vi "Draw.vi"(8 "error in (no error)":errorcluster, 11 "Game Data in":T1) -> (0 "error out":errorcluster, 2 "Colors":u32[](array[colorbox]), 3 "Game Data out":T1)   [LabVIEW 2025]
uses:
  Game Data.ctl
  Bullet Data.ctl
  Game State.ctl
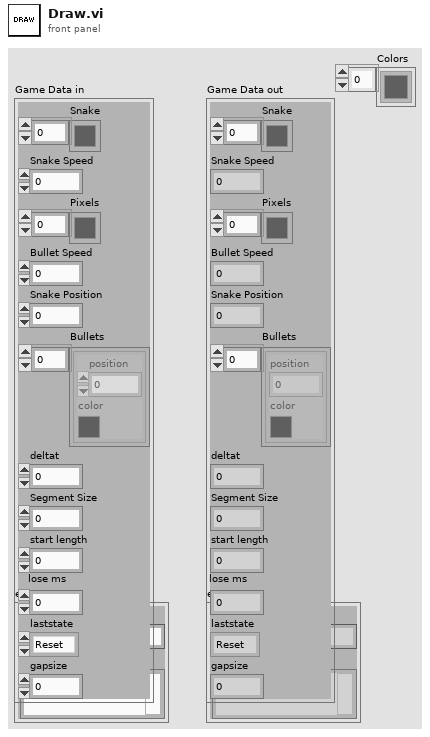
[diagram p1: front panel]
types:
  T1 = typedef "Game Data.ctl" = cluster{"Snake":u32[], "Snake Speed":dbl, "Pixels":u32[], "Bullet Speed":dbl, "Snake Position":dbl, "Bullets":T2[], "deltat":dbl, "Segment Size":dbl, "start length":u32, "lose ms":u32, "laststate":T3, "gapsize":i32}
  T2 = typedef "Bullet Data.ctl" = cluster{"position":dbl, "color":u32}
  T3 = typedef "Game State.ctl" = enum16{"Reset", "Idle", "Start", "Playing", "Win", "Lose"}
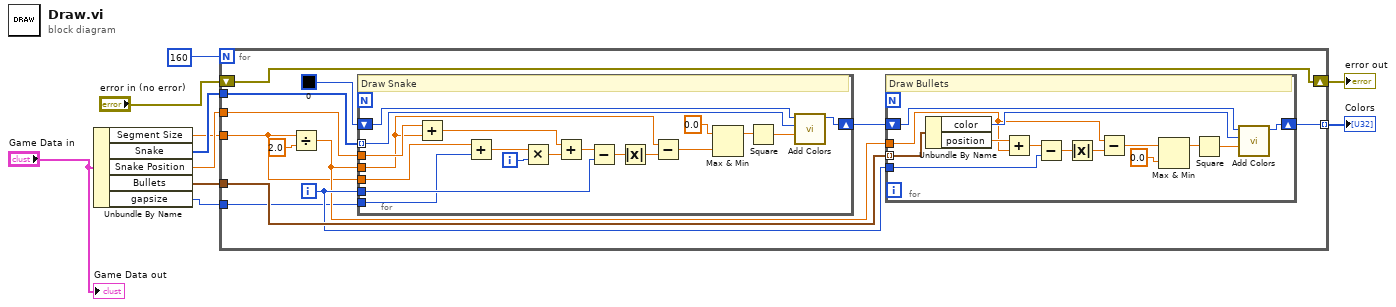
[diagram p0: block diagram]
diagram:
  n1 = Unbundle By Name("Game Data in") -> ("Segment Size"=w4:dbl, "Snake"=w6:u32[], "Snake Position"=w5:dbl, "Bullets"=w7:T2[], "gapsize"=w1:i32)
  n2 = for {
    N: 160 ("dimension size") -> [_]
    shift-right: [w22] -> w8
    shift-left: "error in (no error)" -> [w22]
    tunnel: w7 -> [w19]
    tunnel: w6 -> [w21]
    tunnel: w5 -> [w20]
    tunnel: [w14] -> w3 mode=indexing
    tunnel: w4 -> [w12]
    tunnel: w1 -> [w11]
    i -> [w18]
    n3 = Divide(x=w12, y=2.0) -> (x/y=w13:dbl)
    n4 = for {
      tunnel: w21 -> [w52] mode=indexing
      tunnel: w13 -> [w40]
      tunnel: w20 -> [w54]
      tunnel: w18 -> [w45]
      shift-right: [w49] -> w15
      shift-left: u32 0 ("Color out") -> [w50]
      tunnel: w12 -> [w42]
      tunnel: w11 -> [w37]
      i -> [w55]
      # "Draw Snake"
      n5 = Add(x=w54, y=w40) -> (x+y=w41:dbl)
      n6 = Add(x=w42, y=w37) -> (x+y=w43:dbl)
      n7 = Multiply(x=w43, y=w55) -> (x*y=w53:dbl)
      n8 = Add(x=w41, y=w53) -> (x+y=w46:dbl)
      n9 = Subtract(x=w46, y=w45) -> (x-y=w44:dbl)
      n10 = Absolute Value(x=w44) -> (abs(x)=w47:dbl)
      n11 = Subtract(x=w40, y=w47) -> (x-y=w51:dbl)
      n12 = Max & Min(x=0.0, y=w51) -> (max(x,y)=w39:dbl)  [unwired: 1 out]
      n13 = Square(x=w39) -> (x^2=w38:dbl)
      n14 = call "Add Colors.vi"("Factor (1)"=w38, "Color in"=w52, "color"=w50) -> ("Color out"=w49:u32)  [unwired: 8 in]
    }
    n15 = for {
      tunnel: w19 -> [w36] mode=indexing
      tunnel: w13 -> [w24]
      tunnel: w18 -> [w34]
      shift-right: [w29] -> w14
      shift-left: w15 -> [w28]
      # "Draw Bullets"
      n16 = Unbundle By Name(w36) -> ("color"=w27:u32, "position"=w35:dbl)
      n17 = Add(x=w35, y=w24) -> (x+y=w25:dbl)
      n18 = Subtract(x=w25, y=w34) -> (x-y=w33:dbl)
      n19 = Absolute Value(x=w33) -> (abs(x)=w32:dbl)
      n20 = Subtract(x=w24, y=w32) -> (x-y=w31:dbl)
      n21 = Max & Min(x=w31, y=0.0) -> (max(x,y)=w26:dbl)  [unwired: 1 out]
      n22 = Square(x=w26) -> (x^2=w23:dbl)
      n23 = call "Add Colors.vi"("Factor (1)"=w23, "Color in"=w27, "color"=w28) -> ("Color out"=w29:u32)  [unwired: 8 in]
    }
  }
  "error out" <- w8
  "Colors" <- w3
  "Game Data out" <- "Game Data in"
